vi "TCP-IP Link.Add Length Header, 3 Chars.vi"(11 "Message":string) -> (3 "Message + Header":string)   [LabVIEW 2024, in "EQMF.lvlib" / "TCP-IP.lvlib"]
uses:
  TCP-IP.lvlib
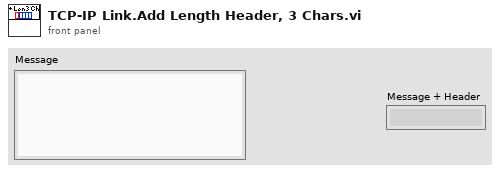
[diagram p1: front panel]
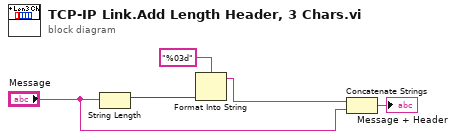
[diagram p0: block diagram]
diagram:
  n1 = String Length(string="Message") -> (length=w2:i32)
  n2 = Format Into String(format string="%03d", w2) -> (resulting string=w1:string)  [unwired: 2 in, 1 out]
  n3 = Concatenate Strings(w1, "Message") -> (→"Message + Header":string)
